vi "Register PPLs.vi"(7 "Show UI?(F)":bool, 8 "error in":errorcluster, 11 "Interrupt":refnum<notifier>) -> (0 "error out":errorcluster, 1 "Success?":bool)   [LabVIEW 2019, in "ClassLoader.lvlib"]
doc: "Scan for unregistered PPLs and cache new PPLs.\nCan be interrupted using the 'Load Interrupt'. Can show a UI."
uses:
  ClassLoader.lvlib
panel:
  out "Active PPL":string
  out "Caching progress":i32(slide) scale=0.0..15.0
  in  "Abort":bool
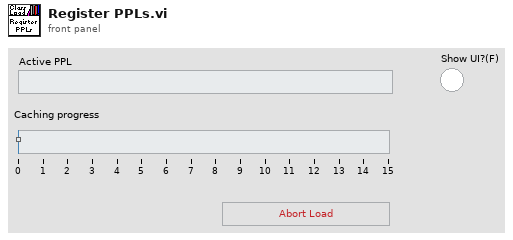
[diagram p1: front panel]
types:
  T1 = enum32{"Invalid", "Standard", "Closed", "Hidden", "Minimized", "Maximized"}
  T2 = typedef "ClassLoader.lvlib/Ctl_PPL Details.ctl" = cluster{"Name":string, "Path":path, "Version":string}
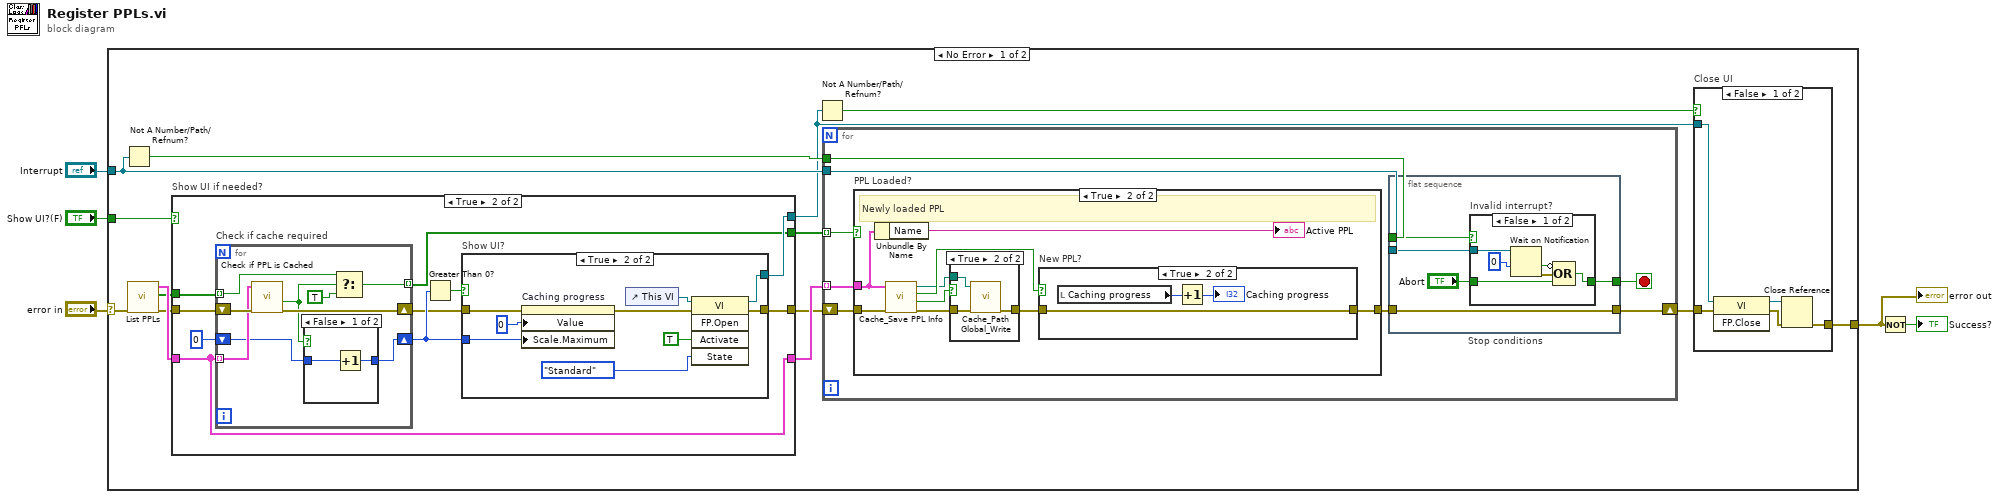
[diagram p0: block diagram]
diagram:
  n1 = case shown="No Error" "error in" {
    selector: "error in" -> [w19 w99]
    tunnel: [w8 w99] -> w2
    tunnel: "Interrupt" -> [w17 _]
    tunnel: "Show UI?(F)" -> [w16 _]
    frame No Error {
      n2 = Not A Number/Path/Refnum?(number/path/refnum=w17) -> (NaN/Path/Refnum?=w18:bool)
      n3 = call "List PPLs.vi"("error in"=w19) -> ("error out"=w13:errorcluster, "Loaded?"=w7:bool[], "PPL Details"=w15:T2[])  [unwired: 8 in]
      n4 = case "Show UI if needed?" shown="True" w16 {
        tunnel: [w28 w37] -> w14
        tunnel: w15 -> [w28 w37]
        tunnel: [w27 w32] -> w12
        tunnel: w13 -> [w27 w38]
        tunnel: [_ w31] -> w10
        tunnel: [w26 w29] -> w6
        tunnel: w7 -> [w26 w30]
        frame False {
        }
        frame True {
          n5 = for "Check if cache required" {
            shift-right: [w56] -> w33
            shift-left: w38 -> [w57]
            tunnel: w37 -> [w55] mode=indexing
            shift-right: [w54] -> w34
            shift-left: 0 -> [w53]
            tunnel: w30 -> [w52] mode=indexing
            tunnel: [w50] -> w29 mode=indexing
            n6 = call "Check if PPL is Cached.vi"("error in"=w57, "PPL Details"=w55) -> ("error out"=w56:errorcluster, "Is Cached?"=w51:bool)  [unwired: 7 in, 1 out]
            n7 = case shown="False" w51 {
              tunnel: [w58 w60] -> w54
              tunnel: w53 -> [w59 w60]
              frame False {
                n8 = Increment(x=w59) -> (x+1=w58:i32)
              }
              frame True {
              }
            }
            n9 = Select(t=w52, s=w51, f=TRUE) -> (s? t:f=w50:bool)
          }
          n10 = Greater Than 0?(x=w34) -> (x > 0?=w35:bool)
          n11 = case "Show UI?" shown="True" w35 {
            tunnel: w34 -> [_ w45]
            tunnel: w33 -> [w39 w43]
            tunnel: [w39 w41] -> w32
            tunnel: [_ w40] -> w31
            frame False {
            }
            frame True {
              n12 = property on="Caching progress" class="Slide (strict)"(error in=w43, "Value"=0 ("Caching progress"), "Scale.Maximum"=w45) -> (error out=w42:errorcluster)  [unwired: 1 in, 1 out]
              n13 = control-ref of="This VI"() -> (w48:refnum<vi>)
              n14 = invoke class="VI" method="FP.Open"(reference=w48, error in=w42, "Activate"=TRUE, "State"=T1."Standard") -> (reference out=w40:refnum<vi>, error out=w41:errorcluster)  [unwired: 1 in, 3 out]
            }
          }
        }
      }
      n15 = Not A Number/Path/Refnum?(number/path/refnum=w10) -> (NaN/Path/Refnum?=w11:bool)
      n16 = for {
        tunnel: w14 -> [w67] mode=indexing
        tunnel: w6 -> [w68] mode=indexing
        shift-right: [w64] -> w9
        shift-left: w12 -> [w66]
        tunnel: w18 -> [w63]
        tunnel: w17 -> [w62]
        stop <- w61 stop-if-true
        n17 = case "PPL Loaded?" shown="True" w68 {
          tunnel: w67 -> [_ w88]
          tunnel: w66 -> [w81 w90]
          tunnel: [w81 w89] -> w65
          frame False {
            # "Previously loaded PPL"
          }
          frame True {
            # "Newly loaded PPL"
            n18 = Unbundle By Name(w88) -> ("Name"=→"Active PPL":string)
            n19 = call "Cache_Save PPL Info.vi"("error in"=w90, "PPL Details"=w88) -> ("error out"=w84:errorcluster, "Success?"=w85:bool, "New Info Loaded?"=w86:bool, "Cache Path"=w82:path)  [unwired: 6 in]
            n20 = case shown="True" w85 {
              tunnel: [w91 w93] -> w83
              tunnel: w84 -> [w91 w92]
              tunnel: w82 -> [_ w94]
              frame False {
              }
              frame True {
                n21 = call "Cache_Path Global_Write.vi"("error in (no error)"=w92, "Cache Path"=w94) -> ("error out"=w93:errorcluster)  [unwired: 7 in, 2 out]
              }
            }
            n22 = case "New PPL?" shown="True" w86 {
              tunnel: [w95 w98] -> w89
              tunnel: w83 -> [w95 w98]
              frame False {
              }
              frame True {
                n23 = local read "Caching progress"() -> (w96:i32)
                n24 = Increment(x=w96) -> (x+1=→"Caching progress":i32)
              }
            }
          }
        }
        n25 = flat-sequence "Stop conditions" {
          tunnel: [w73] -> w64
          tunnel: w65 -> [w73]
          tunnel: w63 -> [w72]
          tunnel: w62 -> [w71]
          tunnel: [w70] -> w61
          frame #0 {
            n26 = case "Invalid interrupt?" shown="False" w72 {
              tunnel: w71 -> [w79 _]
              tunnel: [w75 w80] -> w70
              tunnel: "Abort" -> [w74 w80]
              frame False {
                n27 = Wait on Notification(notifier=w79, timeout in ms (-1)=0) -> (timed out?=w76:bool, error out=w77:errorcluster)  [unwired: 2 in, 2 out]
                n28 = Compound Arithmetic op=OR(invert w76, w77, w74) -> (w75:bool)
              }
              frame True {
              }
            }
          }
        }
      }
      n29 = case "Close UI" shown="False" w11 {
        tunnel: w10 -> [w24 _]
        tunnel: w9 -> [w23 w25]
        tunnel: [w20 w25] -> w8
        frame False {
          n30 = invoke class="VI" method="FP.Close"(reference=w24, error in=w23) -> (reference out=w21:refnum<vi>, error out=w22:errorcluster)  [unwired: 1 in, 1 out]
          n31 = Close Reference(reference=w21, error in (no error)=w22) -> (error out=w20:errorcluster)
        }
        frame True {
        }
      }
    }
    frame Error {
    }
  }
  "error out" <- w2
  n32 = Not(x=w2) -> (.not. x?=→"Success?":bool)
